vi "XL320_Query Temperature.vi"(8 "error in":errorcluster, 10 "Motor ID (0)":u8, 11 "VISA resource name":refnum<visa-resource-name>) -> (0 "error out":errorcluster, 2 "Temperature (C)":u8(slide) scale=0.0..150.0, 3 "VISA resource name out":refnum<visa-resource-name>)   [LabVIEW 2017, in "Dynamixel XL320.lvlib"]
doc: "Retrieves the motor's temperature."
uses:
  <instrlib>/Dynamixel XL320 (Drivers instrument)/Dynamixel XL320.lvlib
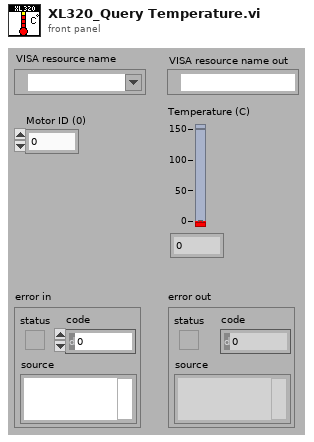
[diagram p1: front panel]
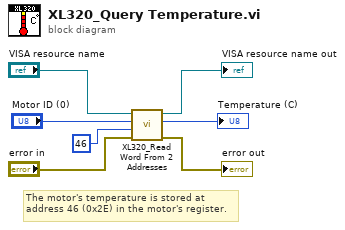
[diagram p0: block diagram]
diagram:
  # "The motor's temperature is stored at \naddress 46 (0x2E) in the motor's register."
  n1 = call <instrlib>:"XL320_Read Word From 2 Addresses.vi"("Error in (no error)"="error in", "Address number (0)"=u8 46 ("Address # DEC"), "Motor ID (0)"="Motor ID (0)", "VISA resource name"="VISA resource name") -> ("error out"=→"error out":errorcluster, "Data"=→"Temperature (C)":u16, "VISA resource name out"=→"VISA resource name out":refnum<visa-resource-name>)  [unwired: 5 in]
